vi "_PC_Daemon_Pref enableObj.vi"(7 "engModeStr":refnum<vi>, 8 "error in (no error)":errorcluster, 11 "tabCtrlRefnum in":refnum<vi>) -> (0 "error out":errorcluster, 3 "tabCtrlRefnum out":refnum<vi>)   [LabVIEW 2018]
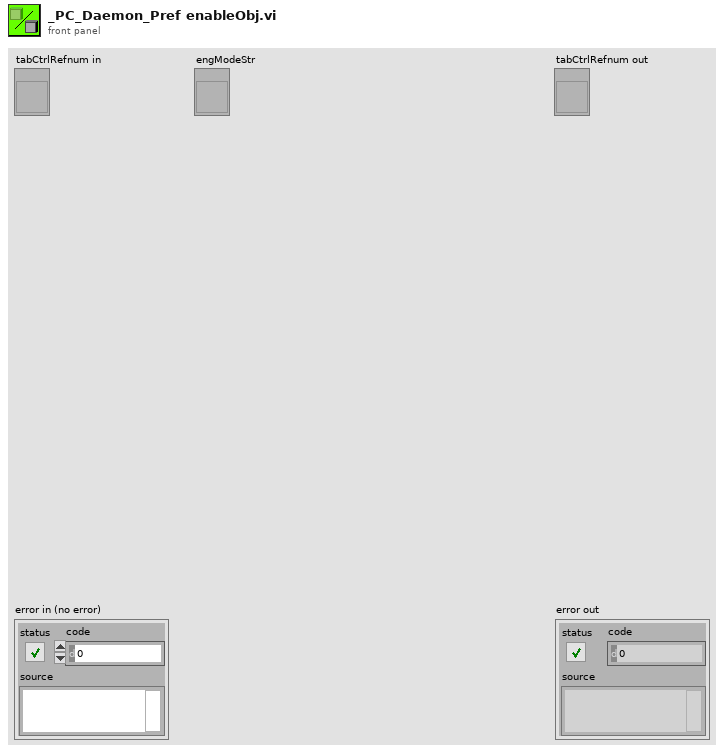
[diagram p1: front panel]
types:
  T1 = enum8{"Enabled", "Disabled", "Disabled and Grayed Out"}
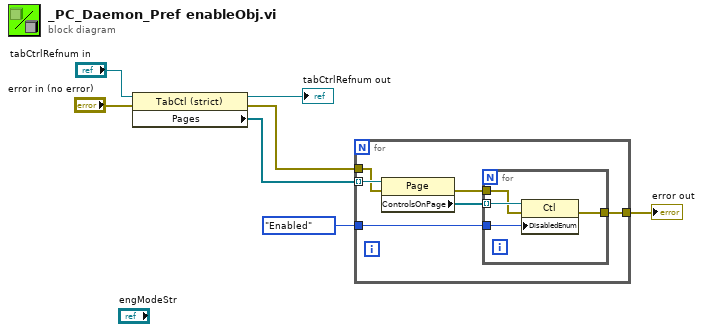
[diagram p0: block diagram]
diagram:
  n1 = property class="TabCtl (strict)"(reference="tabCtrlRefnum in", error in="error in (no error)") -> (reference out=→"tabCtrlRefnum out":refnum<vi>, error out=w7:errorcluster, "Pages"=w6:refnum<vi>[])
  n2 = for {
    tunnel: w6 -> [w13] mode=indexing
    tunnel: T1."Enabled" ("Disabled") -> [w12]
    tunnel: [w10] -> w3
    tunnel: w7 -> [w8]
    n3 = property class="Page"(reference=w13, error in=w8) -> (error out=w9:errorcluster, "ControlsOnPage"=w11:refnum<vi>[])  [unwired: 1 out]
    n4 = for {
      tunnel: w11 -> [w17] mode=indexing
      tunnel: w12 -> [w16]
      tunnel: [w15] -> w10
      tunnel: w9 -> [w14]
      n5 = property class="Ctl"(reference=w17, error in=w14, "DisabledEnum"=w16) -> (error out=w15:errorcluster)  [unwired: 1 out]
    }
  }
  "error out" <- w3
